vi "Main.vi"() -> ()   [LabVIEW 2021]
doc: "Use this template to build a simple state machine design pattern. Each state executes code and determines which state to transition to."
uses:
  Controls/State.ctl
  Controls/Data.ctl
  Controls/Toggle Channel.ctl
  Controls/Script Trigger Routing.ctl
  <vilib>/regexp/Match Regular Expression.xnode
  Controls/Debugging Checklist.ctl
panel:
  out "Debugging Checklist":T1
  in  "Tab Control":T2(tab)
  in  "Start Chn1 First?":bool
  in  "FGEN Resource Name":refnum<k15>
  in  "Sample Rate":dbl=20000000.0 caption="Sample Rate (Hz)" format="%#_6p"
  in  "Save Wfm List":bool
  in  "Load Wfm List":bool
  out "Waveform Preview":dbl[](graph)
  in  "Add Standard Wfm":bool
  in  "Add Custom Wfm":bool
  in  "Waveform List":i32(listbox)
  in  "Delete Selected Wfm":bool
  in  "Rename Selected Wfm":bool
  out "Total Variables":i32
  in  "Script Variable List":string[][](table) caption="Script Variable List (Editable)"
  in  "Script Trigger Routings":T3[](array[typedef])
  in  "Save Variable List":bool
  in  "Load Variable List":bool
  in  "Size to Duration":bool
  in  "Duration to Size":bool
  in  "Copy Sample Size":bool
  in  "Copy Duration":bool
  in  "Sample Size":i32
  in  "Duration (s)":dbl format="%#_6p"
  in  "Toggle Channels":T4[](array[typedef]) {"Initial State" items=["High"=101, "Low"=102]}
  in  "Start":bool
  in  "Stop":bool
  in  "Chn1 Script":string="script myScript2\n  Wait until scriptTrigger0\n  Generate Sine1kHz100us\n  Generate DcOff10us\nend script" caption="Script"
  in  "Chn0 Script":string="script myScript1\n  Generate DcOff10us\n  Generate DcOn120us marker0(tON1, tOFF1) marker1(tON2, tOFF2)\n  Generate DcOff10us\nend script" caption="Script"
  in  "Exit":bool
  # "FGEN Dual-Channel Scripts Mode Panel"
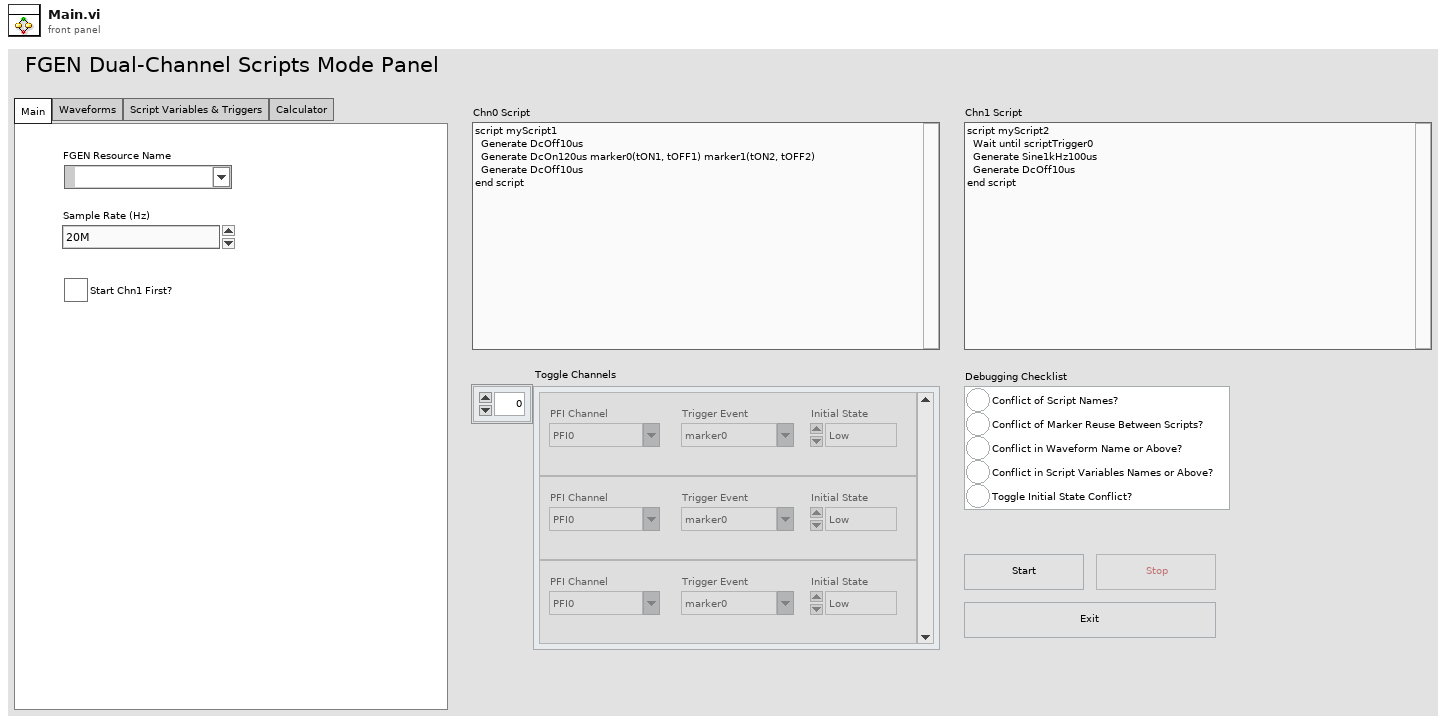
[diagram p1: front panel]
types:
  T1 = typedef "Debugging Checklist.ctl" = cluster{"Conflict of Script Names?":bool, "Conflict of Marker Reuse Between Scripts?":bool, "Conflict in Waveform Name or Above?":bool, "Conflict in Script Variables Names or Above?":bool, "Toggle Initial State Conflict?":bool}
  T2 = enum32{"Main", "Waveforms", "Script Variables & Triggers", "Calculator"}
  T3 = typedef "Script Trigger Routing.ctl" = cluster{"ID":string, "Trigger Source":string}
  T4 = typedef "Toggle Channel.ctl" = cluster{"PFI Channel":string, "Trigger Event":string, "Initial State":u16}
  T5 = typedef "Data.ctl" = cluster{"FGEN Resource Name":refnum<k15>, "Sample Rate":dbl, "Start Chn1 First?":bool, "Script Trigger Routings":T3[], "Chn0 Script":string, "Chn1 Script":string, "Toggle Channels":T4[], "Script Variable List":string[][], "Session Initialized?":bool, "Original Waveforms":waveform(dbl)[], "Chn0 Script Name":string, "Chn1 Script Name":string}
  T6 = typedef "State.ctl" = enum16{"Initialize", "Update Sample Rate", "Update Waveform List", "Update Script Variable List", "Update Scripts", "Update Toggle Channels", "Debugging Checklist", "Wait for Event", "Prepare", "Start", "Running", "Stop", "Handle Error", "Exit"}
  T7 = enum8{"Enabled", "Disabled", "Disabled and Grayed Out"}
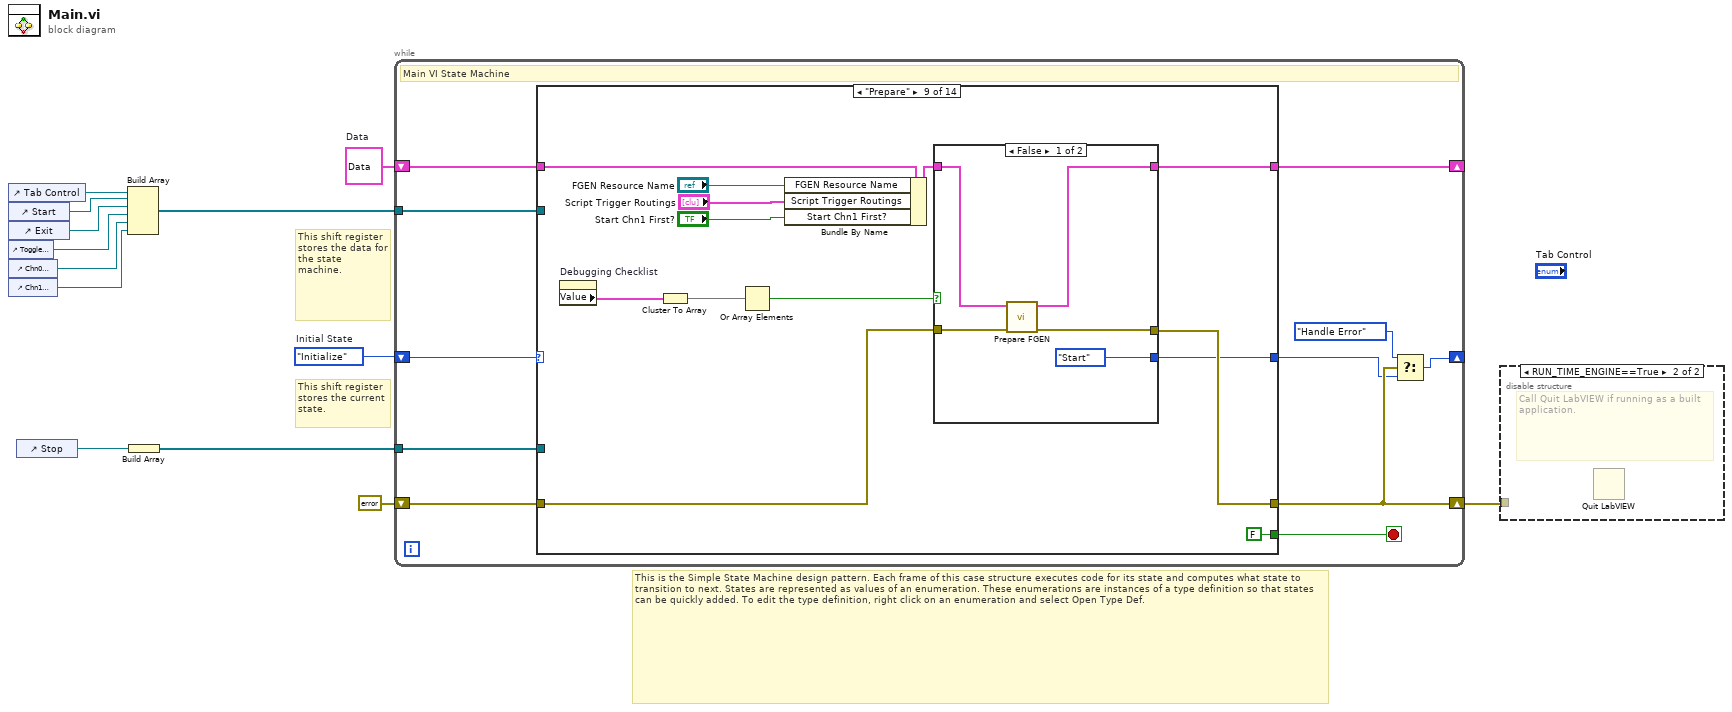
[diagram p0: block diagram]
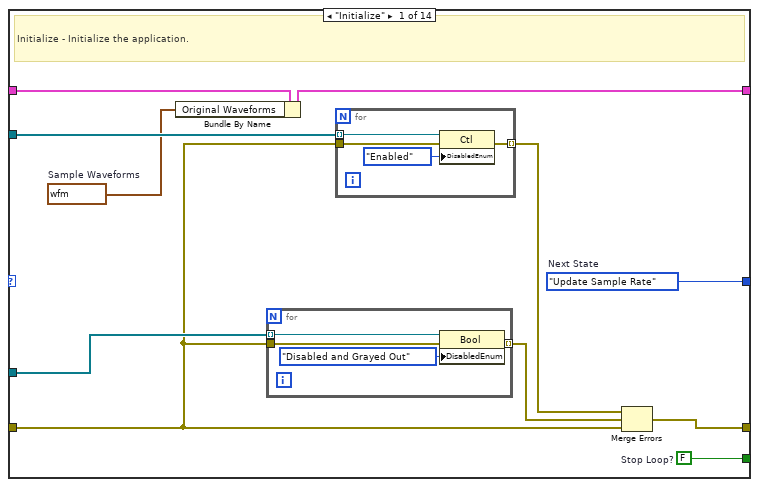
[diagram p3: hidden frame]
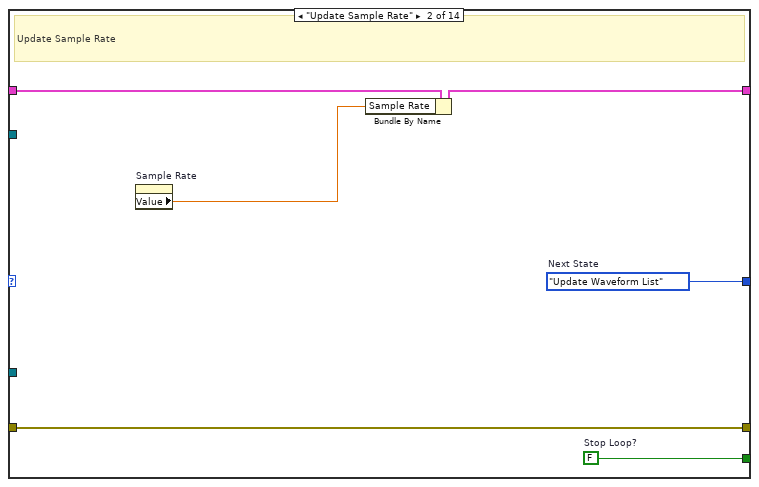
[diagram p4: hidden frame]
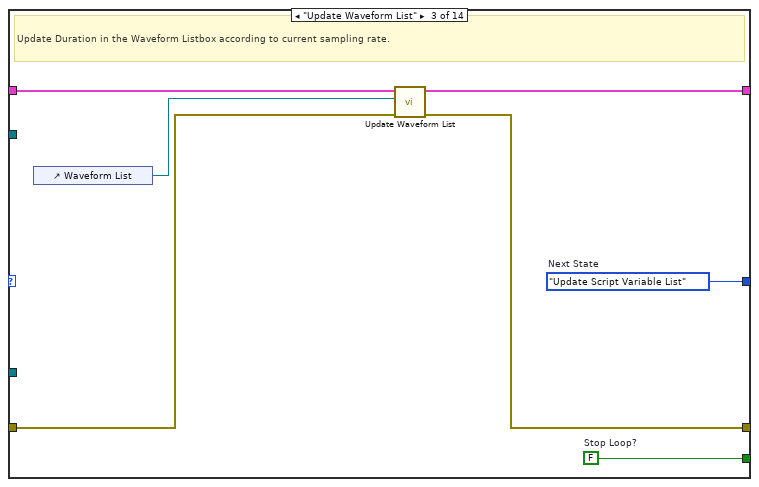
[diagram p5: hidden frame]
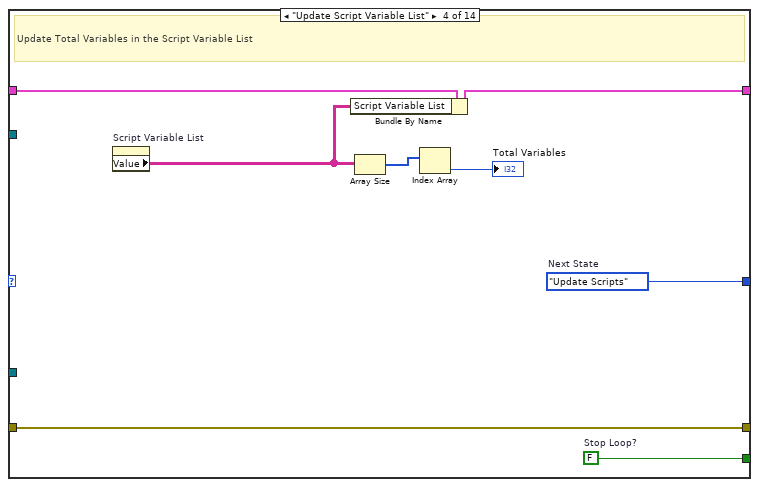
[diagram p6: hidden frame]
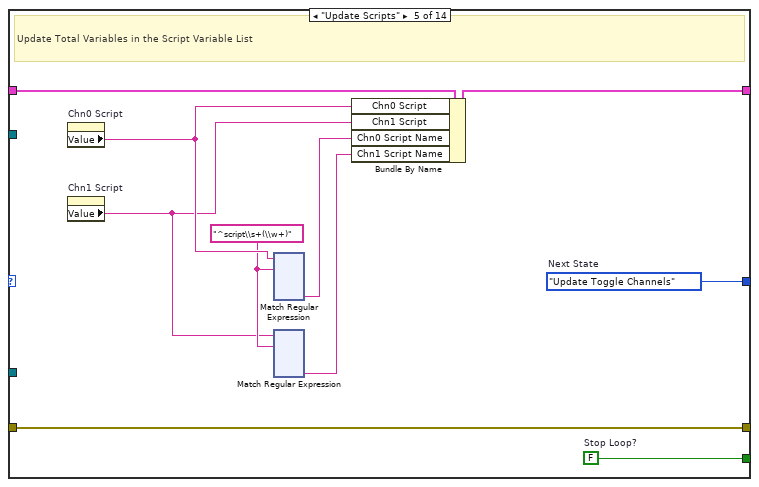
[diagram p7: hidden frame]
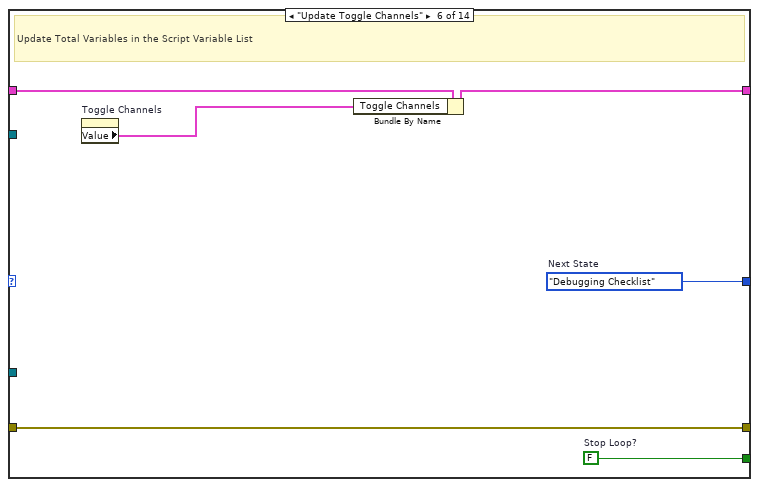
[diagram p8: hidden frame]
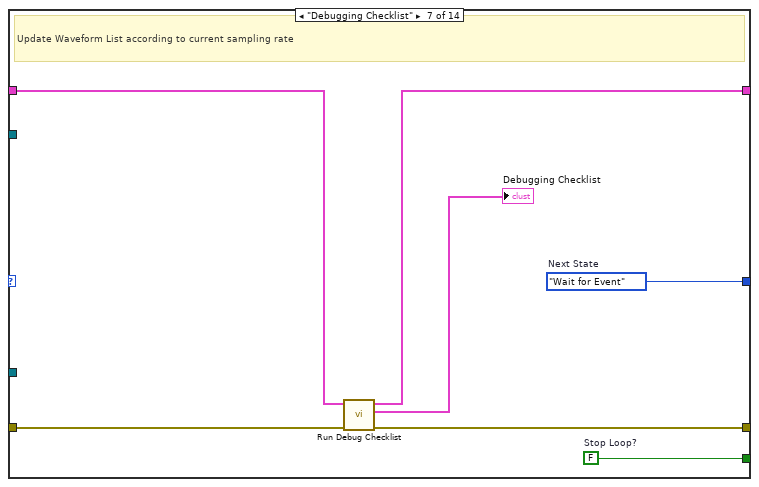
[diagram p9: hidden frame]
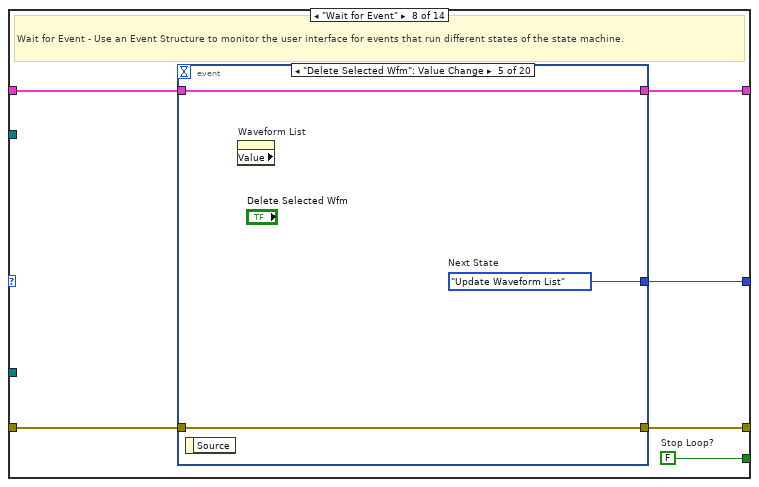
[diagram p10: hidden frame]
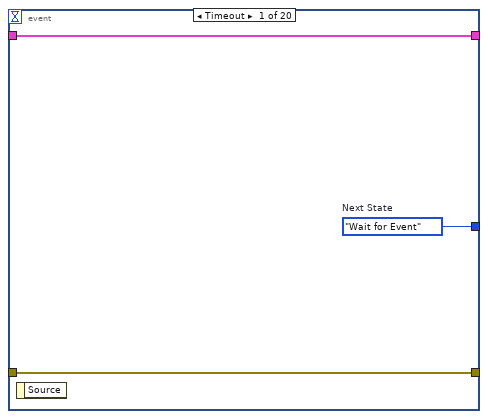
[diagram p11: hidden frame]
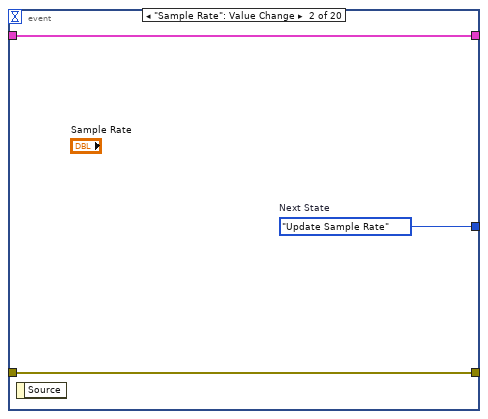
[diagram p12: hidden frame]
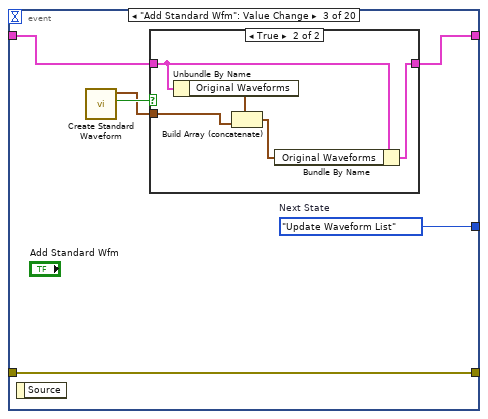
[diagram p13: hidden frame]
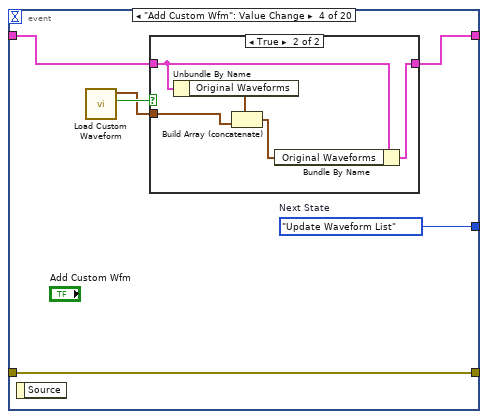
[diagram p15: hidden frame]
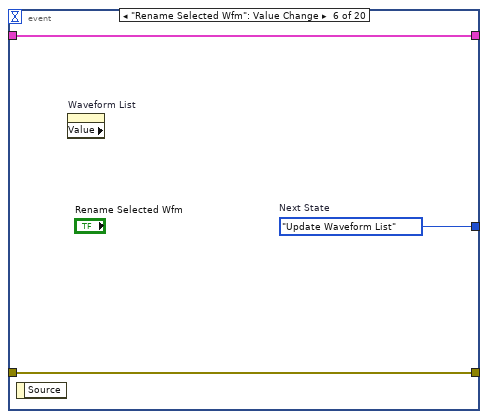
[diagram p17: hidden frame]
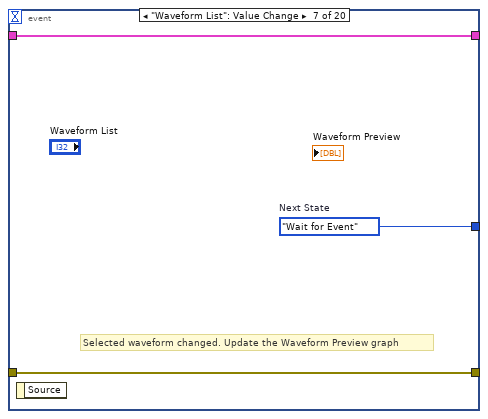
[diagram p18: hidden frame]
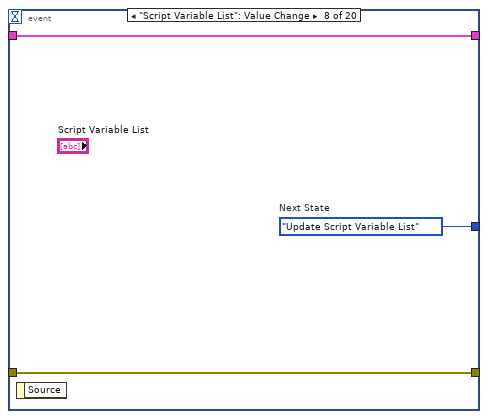
[diagram p19: hidden frame]
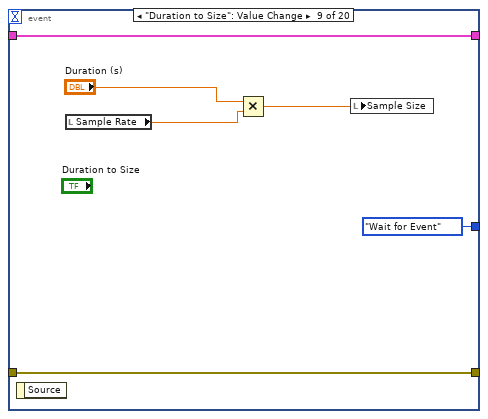
[diagram p20: hidden frame]
diagram:
  w12 = T5 {"FGEN Resource Name"="", "Sample Rate"=0.0, "Start Chn1 First?"=FALSE, "Script Trigger Routings"=[], "Chn0 Script"="", "Chn1 Script"="", "Toggle Channels"=[], "Script Variable List"=[], "Session Initialized?"=FALSE, "Original Waveforms"=[], "Chn0 Script Name"="", "Chn1 Script Name"=""}  # Data
  w13 = State."Initialize"  # Initial State
  # "This shift register stores the data for the state machine."
  # "This is the Simple State Machine design pattern. Each frame of this case structure executes code for its state and computes what state to transition to next. States are represented as values of an enumeration. These enumerations are instances of a type definition so that states can be quickly added. To edit the type definition, right click on an enumeration and select Open Type Def."
  # "This shift register stores the current state."
  n1 = control-ref of="Tab Control"() -> (w9:refnum<vi>)
  n2 = control-ref of="Start"() -> (w8:refnum<vi>)
  n3 = control-ref of="Exit"() -> (w7:refnum<vi>)
  n4 = control-ref of="Toggle Channels"() -> (w6:refnum<vi>)
  n5 = control-ref of="Chn0 Script"() -> (w5:refnum<vi>)
  n6 = control-ref of="Chn1 Script"() -> (w4:refnum<vi>)
  n7 = control-ref of="Stop"() -> (w3:refnum<vi>)
  n8 = Build Array(w9, w8, w7, w6, w5, w4) -> (w2:refnum<vi>[])
  n9 = Build Array(w3) -> (w1:refnum<vi>[])
  n10 = while {
    shift-right: [w20] -> _
    shift-left: w13 -> [w16]
    shift-right: [w23] -> _
    shift-left: w12 -> [w24]
    shift-right: [w19] -> w10
    shift-left: errorcluster {"status"=FALSE, "code"=0, "source"=""} ("error constant") -> [w22]
    tunnel: w2 -> [w14]
    tunnel: w1 -> [w15]
    stop <- w21 stop-if-true
    # "Main VI State Machine"
    n11 = case shown="\"Prepare\"" w16 {
      tunnel: [w35 w49 w56 w64 w74 w318 w325 w331 w423 State."Running" w470 State."Wait for Event" w496 w501] -> w17
      tunnel: [w34 w48 w55 w63 w73 w317 w324 w330 FALSE ("Stop Loop?") FALSE ("Stop Loop?") FALSE ("Stop Loop?") FALSE ("Stop Loop?") FALSE ("Stop Loop?") w500] -> w21
      tunnel: w24 -> [w33 w47 w52 w62 w72 w316 w320 w329 w434 w445 w465 w474 w494 w498]
      tunnel: [w26 w45 w51 w60 w70 w314 w321 w328 w432 w444 w464 w473 w494 w498] -> w23
      tunnel: w22 -> [w27 w46 w54 w61 w71 w315 w323 w327 w422 w450 w472 w479 w493 w499]
      tunnel: [w30 w46 w53 w61 w71 w315 w322 w326 w431 w449 w466 w478 w491 w499] -> w19
      tunnel: w15 -> [w31 _ _ _ _ _ _ _ _ w451 _ w480 _ _]
      tunnel: w14 -> [w32 _ _ _ _ _ _ _ _ w452 _ w481 _ _]
      frame "Initialize" {
        w25 = waveform(dbl)[] [{"t0"=timestamp(0 s since 1904-01-01), "dt"=1e-06, "Y"=[0.0, 0.0, 0.0, 0.0, 0.0, 0.0, 0.0, 0.0, 0.0, 0.0], "attributes"=variant("NI_ChannelName"=variant(string "DcOff10us"), "NI_ExpIsRelativeTime"=variant(bool TRUE), "NI_ExpStartTimeStamp"=variant(timestamp timestamp(3848638021.4949055 s since 1904-01-01)), "NI_ExpTimeStamp"=variant(timestamp timestamp(3848638021.4949055 s since 1904-01-01)), "NI_ExpXDimension"=variant(string "t"))}, {"t0"=timestamp(0 s since 1904-01-01), "dt"=1e-06, "Y"=[1.0, 1.0, 1.0, 1.0, 1.0, 1.0, 1.0, 1.0, 1.0, 1.0, 1.0, 1.0, 1.0, 1.0, 1.0, 1.0, 1.0, 1.0, 1.0, 1.0, 1.0, 1.0, 1.0, 1.0, 1.0, 1.0, 1.0, 1.0, 1.0, 1.0, 1.0, 1.0, 1.0, 1.0, 1.0, 1.0, 1.0, 1.0, 1.0, 1.0, 1.0, 1.0, 1.0, 1.0, 1.0, 1.0, 1.0, 1.0, 1.0, 1.0, 1.0, 1.0, 1.0, 1.0, 1.0, 1.0, 1.0, 1.0, 1.0, 1.0, 1.0, 1.0, 1.0, 1.0, 1.0, 1.0, 1.0, 1.0, 1.0, 1.0, 1.0, 1.0, 1.0, 1.0, 1.0, 1.0, 1.0, 1.0, 1.0, 1.0, 1.0, 1.0, 1.0, 1.0, 1.0, 1.0, 1.0, 1.0, 1.0, 1.0, 1.0, 1.0, 1.0, 1.0, 1.0, 1.0, 1.0, 1.0, 1.0, 1.0, 1.0, 1.0, 1.0, 1.0, 1.0, 1.0, 1.0, 1.0, 1.0, 1.0, 1.0, 1.0, 1.0, 1.0, 1.0, 1.0, 1.0, 1.0, 1.0, 1.0], "attributes"=variant("NI_ChannelName"=variant(string "DcOn120us"), "NI_ExpIsRelativeTime"=variant(bool TRUE), "NI_ExpStartTimeStamp"=variant(timestamp timestamp(3848638021.4959054 s since 1904-01-01)), "NI_ExpTimeStamp"=variant(timestamp timestamp(3848638021.4959054 s since 1904-01-01)), "NI_ExpXDimension"=variant(string "t"))}, {"t0"=timestamp(0 s since 1904-01-01), "dt"=5e-08, "Y"=array[2000 elements], "attributes"=variant("NI_ChannelName"=variant(string "Sine1kHz100us"), "NI_ExpIsRelativeTime"=variant(bool TRUE), "NI_ExpStartTimeStamp"=variant(timestamp timestamp(3848638021.493907 s since 1904-01-01)), "NI_ExpTimeStamp"=variant(timestamp timestamp(3848638021.493907 s since 1904-01-01)), "NI_ExpXDimension"=variant(string "t"))}]  # Sample Waveforms
        w34 = FALSE  # Stop Loop?
        w35 = State."Update Sample Rate"  # Next State
        # "Initialize - Initialize the application."
        n12 = Bundle By Name(cluster=w33, "Original Waveforms"=w25) -> (w26:T5)
        n13 = for {
          tunnel: w31 -> [w38] mode=indexing
          tunnel: [w37] -> w29 mode=indexing
          tunnel: w27 -> [w36]
          n14 = property on="Property Node" class="Bool"(reference=w38, error in=w36, "DisabledEnum"=T7."Disabled and Grayed Out" ("Disabled")) -> (error out=w37:errorcluster)  [unwired: 1 out]
        }
        n15 = for {
          tunnel: w32 -> [w42] mode=indexing
          tunnel: [w41] -> w28 mode=indexing
          tunnel: w27 -> [w40]
          n16 = property on="Property Node" class="Ctl"(reference=w42, error in=w40, "DisabledEnum"=T7."Enabled" ("Disabled")) -> (error out=w41:errorcluster)  [unwired: 1 out]
        }
        n17 = Merge Errors(w28, w29, w27) -> (w30:errorcluster)
      }
      frame "Update Sample Rate" {
        w48 = FALSE  # Stop Loop?
        w49 = State."Update Waveform List"  # Next State
        # "Update Sample Rate"
        n18 = property on="Sample Rate" class="DigNum (strict)"() -> ("Value"=w44:dbl)  [unwired: 2 in, 2 out]
        n19 = Bundle By Name(cluster=w47, "Sample Rate"=w44) -> (w45:T5)
      }
      frame "Update Waveform List" {
        w55 = FALSE  # Stop Loop?
        w56 = State."Update Script Variable List"  # Next State
        # "Update Duration in the Waveform Listbox according to current sampling rate."
        n20 = control-ref of="Waveform List"() -> (w50:refnum<vi>)
        n21 = call "Update Waveform List.vi"("error in (no error)"=w54, "Waveform Listbox Ref"=w50, "Data In"=w52) -> ("error out"=w53:errorcluster, "Data Out"=w51:T5)  [unwired: 7 in]
      }
      frame "Update Script Variable List" {
        w63 = FALSE  # Stop Loop?
        w64 = State."Update Scripts"  # Next State
        # "Update Total Variables in the Script Variable List"
        n22 = property on="Script Variable List" class="Tbl (strict)"() -> ("Value"=w59:string[][])  [unwired: 2 in, 2 out]
        n23 = Bundle By Name(cluster=w62, "Script Variable List"=w59) -> (w60:T5)
        n24 = Array Size(array=w59) -> (size(s)=w58:i32[])
        n25 = Index Array(array=w58) -> (element=→"Total Variables":i32)  [unwired: 1 in]
      }
      frame "Update Scripts" {
        w67 = "^script\\s+(\\w+)" ("regular expression")
        w73 = FALSE  # Stop Loop?
        w74 = State."Update Toggle Channels"  # Next State
        # "Update Total Variables in the Script Variable List"
        n26 = property on="Chn0 Script" class="Str"() -> ("Value"=w69:string)  [unwired: 2 in, 2 out]
        n27 = property on="Chn1 Script" class="Str"() -> ("Value"=w66:string)  [unwired: 2 in, 2 out]
        n28 = xnode "Match Regular Expression"("input string"=w69, "regular expression"=w67) -> ("submatch 1"=w68:string)  [unwired: 4 in, 5 out]
        n29 = xnode "Match Regular Expression"("input string"=w66, "regular expression"=w67) -> ("submatch 1"=w65:string)  [unwired: 4 in, 5 out]
        n30 = Bundle By Name(cluster=w72, "Chn0 Script"=w69, "Chn1 Script"=w66, "Chn0 Script Name"=w68, "Chn1 Script Name"=w65) -> (w70:T5)
      }
      frame "Update Toggle Channels" {
        w317 = FALSE  # Stop Loop?
        w318 = State."Debugging Checklist"  # Next State
        # "Update Total Variables in the Script Variable List"
        n31 = property on="Toggle Channels" class="Arr (strict)"() -> ("Value"=w313:T4[])  [unwired: 2 in, 2 out]
        n32 = Bundle By Name(cluster=w316, "Toggle Channels"=w313) -> (w314:T5)
      }
      frame "Debugging Checklist" {
        w324 = FALSE  # Stop Loop?
        w325 = State."Wait for Event"  # Next State
        # "Update Waveform List according to current sampling rate"
        n33 = call "Run Debug Checklist.vi"("error in (no error)"=w323, "Data In"=w320) -> ("error out"=w322:errorcluster, "Debugging Checklist"=→"Debugging Checklist":T1, "Data Out"=w321:T5)  [unwired: 7 in]
      }
      frame "Wait for Event" {
        w330 = FALSE  # Stop Loop?
        # "Wait for Event - Use an Event Structure to monitor the user interface for events that run different states of the state machine."
        n34 = event shown="[4] \"Delete Selected Wfm\": Value Change" {
          selector: _ -> [_ _ _ _ _ _ _ _ _ _ _ _ _ _ _ _ _ _ _ _]
          dyn-events: _ -> [_ _ _ _ _ _ _ _ _ _ _ _ _ _ _ _ _ _ _ _]
          timeout: _ -> [_ _ _ _ _ _ _ _ _ _ _ _ _ _ _ _ _ _ _ _]
          tunnel: [w332 w335 w342 w354 w362 w365 w368 w371 State."Wait for Event" ("Next State") State."Wait for Event" ("Next State") State."Wait for Event" ("Next State") State."Wait for Event" ("Next State") State."Debugging Checklist" ("Next State") State."Debugging Checklist" ("Next State") State."Update Waveform List" ("Next State") State."Wait for Event" ("Next State") State."Update Script Variable List" ("Next State") State."Wait for Event" ("Next State") State."Prepare" ("Next State") w421] -> w331
          tunnel: w329 -> [w334 w337 w341 w353 w364 w367 w370 w373 w379 w385 w391 w397 w400 w403 w406 w409 w412 w415 w418 w420]
          tunnel: [w334 w337 w340 w352 w364 w367 w370 w373 w379 w385 w391 w397 w400 w403 w406 w409 w412 w415 w418 w420] -> w328
          tunnel: w327 -> [w333 w336 w343 w355 w363 w366 w369 w372 w378 w384 w390 w396 w399 w402 w405 w408 w411 w414 w417 w419]
          tunnel: [w333 w336 w343 w355 w363 w366 w369 w372 w378 w384 w390 w396 w399 w402 w405 w408 w411 w414 w417 w419] -> w326
          event Timeout {
            w332 = State."Wait for Event"  # Next State
            n35 = event-data() -> ()  [unwired: 1 in, 1 out]
          }
          event "Sample Rate": Value Change {
            w335 = State."Update Sample Rate"  # Next State
            n36 = event-data() -> ()  [unwired: 1 in, 1 out]
          }
          event "Add Standard Wfm": Value Change {
            w342 = State."Update Waveform List"  # Next State
            n37 = event-data() -> ()  [unwired: 1 in, 1 out]
            n38 = call "Create Standard Waveform.vi"() -> ("Waveform Created?"=w339:bool, "Output Waveform"=w338:waveform(dbl))  [unwired: 10 in]
            n39 = case shown="True" w339 {
              tunnel: w341 -> [w344 w349]
              tunnel: [w344 w345] -> w340
              tunnel: w338 -> [_ w347]
              frame False {
              }
              frame True {
                n40 = Unbundle By Name(w349) -> ("Original Waveforms"=w348:waveform(dbl)[])
                n41 = Build Array (concatenate)(w348, w347) -> (w346:waveform(dbl)[])
                n42 = Bundle By Name(cluster=w349, "Original Waveforms"=w346) -> (w345:T5)
              }
            }
          }
          event "Add Custom Wfm": Value Change {
            w354 = State."Update Waveform List"  # Next State
            n43 = event-data() -> ()  [unwired: 1 in, 1 out]
            n44 = call "Load Custom Waveform.vi"() -> ("Waveform Created?"=w351:bool, "Output Waveform"=w350:waveform(dbl))  [unwired: 10 in]
            n45 = case shown="True" w351 {
              tunnel: w353 -> [w356 w361]
              tunnel: [w356 w357] -> w352
              tunnel: w350 -> [_ w359]
              frame False {
              }
              frame True {
                n46 = Unbundle By Name(w361) -> ("Original Waveforms"=w360:waveform(dbl)[])
                n47 = Build Array (concatenate)(w360, w359) -> (w358:waveform(dbl)[])
                n48 = Bundle By Name(cluster=w361, "Original Waveforms"=w358) -> (w357:T5)
              }
            }
          }
          event "Delete Selected Wfm": Value Change {
            w362 = State."Update Waveform List"  # Next State
            n49 = event-data() -> ()  [unwired: 1 in, 1 out]
            n50 = property on="Waveform List" class="MCListbox (strict)" props=["Value"]() -> ()  [unwired: 2 in, 3 out]
          }
          event "Rename Selected Wfm": Value Change {
            w365 = State."Update Waveform List"  # Next State
            n51 = event-data() -> ()  [unwired: 1 in, 1 out]
            n52 = property on="Waveform List" class="MCListbox (strict)" props=["Value"]() -> ()  [unwired: 2 in, 3 out]
          }
          event "Waveform List": Value Change {
            w368 = State."Wait for Event"  # Next State
            # "Selected waveform changed. Update the Waveform Preview graph"
            n53 = event-data() -> ()  [unwired: 1 in, 1 out]
          }
          event "Script Variable List": Value Change {
            w371 = State."Update Script Variable List"  # Next State
            n54 = event-data() -> ()  [unwired: 1 in, 1 out]
          }
          event "Duration to Size": Value Change {
            n55 = event-data() -> ()  [unwired: 1 in, 1 out]
            n56 = local read "Sample Rate"() -> (w375:dbl)
            n57 = Multiply(x="Duration (s)", y=w375) -> (x*y=w374:dbl)
            n58 = local write "Sample Size"(w374) -> ()
          }
          event "Size to Duration": Value Change {
            n59 = event-data() -> ()  [unwired: 1 in, 1 out]
            n60 = local read "Sample Rate"() -> (w382:dbl)
            n61 = Divide(x="Sample Size", y=w382) -> (x/y=w381:dbl)
            n62 = local write "Duration (s)"(w381) -> ()
          }
          event "Copy Duration": Value Change {
            n63 = event-data() -> ()  [unwired: 1 in, 1 out]
            n64 = local read "Duration (s)"() -> (w389:dbl)
            n65 = Format Into String(format string="%#_6p", w389) -> (resulting string=w388:string)  [unwired: 2 in, 1 out]
            n66 = invoke class="App" method="Clipboard.Write"("Param 0"=w388) -> ()  [unwired: 3 in, 4 out]
          }
          event "Copy Sample Size": Value Change {
            n67 = event-data() -> ()  [unwired: 1 in, 1 out]
            n68 = local read "Sample Size"() -> (w395:i32)
            n69 = Format Into String(format string="%d", w395) -> (resulting string=w394:string)  [unwired: 2 in, 1 out]
            n70 = invoke class="App" method="Clipboard.Write"("Param 0"=w394) -> ()  [unwired: 3 in, 4 out]
          }
          event "Chn0 Script", "Chn1 Script": Value Change {
            n71 = event-data() -> ()  [unwired: 1 in, 1 out]
          }
          event "Toggle Channels": Value Change {
            n72 = event-data() -> ()  [unwired: 1 in, 1 out]
          }
          event "Load Wfm List": Value Change {
            n73 = event-data() -> ()  [unwired: 1 in, 1 out]
          }
          event "Save Wfm List": Value Change {
            n74 = event-data() -> ()  [unwired: 1 in, 1 out]
          }
          event "Load Variable List": Value Change {
            n75 = event-data() -> ()  [unwired: 1 in, 1 out]
          }
          event "Save Variable List": Value Change {
            n76 = event-data() -> ()  [unwired: 1 in, 1 out]
          }
          event "Start": Value Change {
            n77 = event-data() -> ()  [unwired: 1 in, 1 out]
          }
          event "Exit": Value Change {
            w421 = State."Exit"  # Next State
            n78 = event-data() -> ()  [unwired: 1 in, 1 out]
          }
        }
      }
      frame "Prepare" {
        n79 = property on="Debugging Checklist" class="Clust (strict)"() -> ("Value"=w426:T1)  [unwired: 2 in, 2 out]
        n80 = Cluster To Array(cluster=w426) -> (array=w425:bool[])
        n81 = Or Array Elements(Boolean array=w425) -> (logical OR=w424:bool)
        n82 = Bundle By Name(cluster=w434, "FGEN Resource Name"="FGEN Resource Name", "Script Trigger Routings"="Script Trigger Routings", "Start Chn1 First?"="Start Chn1 First?") -> (w430:T5)
        n83 = case shown="False" w424 {
          tunnel: [w439 w440] -> w432
          tunnel: w422 -> [w438 w441]
          tunnel: [w437 w441] -> w431
          tunnel: w430 -> [w436 w440]
          tunnel: [State."Start" State."Wait for Event"] -> w423
          frame False {
            n84 = call "Prepare FGEN.vi"("error in (no error)"=w438, "Data In"=w436) -> ("error out"=w437:errorcluster, "Data Out"=w439:T5)  [unwired: 8 in]
          }
          frame True {
            n85 = One Button Dialog(message="Please check the Debug Checklist and fix the issue.") -> ()  [unwired: 1 in, 1 out]
          }
        }
      }
      frame "Start" {
        n86 = call "Start FGEN.vi"("error in (no error)"=w450, "Data In"=w445) -> ("error out"=w446:errorcluster, "Data Out"=w444:T5)  [unwired: 8 in]
        n87 = for {
          tunnel: w452 -> [w457] mode=indexing
          tunnel: w446 -> [w456]
          tunnel: [w455] -> w447 mode=indexing
          n88 = property on="Property Node" class="Ctl"(reference=w457, error in=w456, "DisabledEnum"=T7."Disabled and Grayed Out" ("Disabled")) -> (error out=w455:errorcluster)  [unwired: 1 out]
        }
        n89 = for {
          tunnel: w451 -> [w460] mode=indexing
          tunnel: [w459] -> w448 mode=indexing
          n90 = property on="Property Node" class="Bool"(reference=w460, "DisabledEnum"=T7."Enabled" ("Disabled")) -> (error out=w459:errorcluster)  [unwired: 1 in, 1 out]
        }
        n91 = Merge Errors(w447, w448, w446) -> (w449:errorcluster)
      }
      frame "Running" {
        # "Running until generation finish or user press Stop."
        n92 = call "Check Running FGEN.vi"("error in (no error)"=w472, "Data In"=w465) -> ("error out"=w466:errorcluster, "Done Generation"=w462:bool, "Data Out"=w464:T5)  [unwired: 7 in]
        n93 = Or(x=w462, y="Stop") -> (x .or. y?=w463:bool)
        n94 = Select(t=State."Stop", s=w463, f=State."Running") -> (s? t:f=w470:T6)
      }
      frame "Stop" {
        # "Stop FGEN if session is initialized"
        n95 = call "Stop FGEN.vi"("error in (no error)"=w479, "Data In"=w474) -> ("error out"=w475:errorcluster, "Data Out"=w473:T5)  [unwired: 8 in]
        n96 = for {
          tunnel: w481 -> [w486] mode=indexing
          tunnel: w475 -> [w485]
          tunnel: [w484] -> w476 mode=indexing
          n97 = property on="Property Node" class="Ctl"(reference=w486, error in=w485, "DisabledEnum"=T7."Enabled" ("Disabled")) -> (error out=w484:errorcluster)  [unwired: 1 out]
        }
        n98 = for {
          tunnel: w480 -> [w489] mode=indexing
          tunnel: [w488] -> w477 mode=indexing
          n99 = property on="Property Node" class="Bool"(reference=w489, "DisabledEnum"=T7."Disabled and Grayed Out" ("Disabled")) -> (error out=w488:errorcluster)  [unwired: 1 in, 1 out]
        }
        n100 = Merge Errors(w476, w477, w475) -> (w478:errorcluster)
      }
      frame "Handle Error" {
        w496 = State."Stop"  # Next State
        # "Display error message and clear it. Stop and close FGEN if needed."
        n101 = call <vilib>:"Simple Error Handler.vi"("error in (no error)"=w493) -> ("error out"=w492:errorcluster)  [unwired: 4 in, 4 out]
        n102 = call <vilib>:"Clear Errors.vi"("error in (no error)"=w492) -> ("error out"=w491:errorcluster)  [unwired: 5 in, 1 out]
      }
      frame "Exit", Default {
        w500 = TRUE  # Stop Loop?
        # "Exit - Exit the application."
        n103 = Unbundle By Name(w498) -> ("Session Initialized?"=w497:bool)
        n104 = case shown="True" w497 {
          tunnel: [State."Stop" State."Exit"] -> w501
          frame True {
            n105 = One Button Dialog(message="Session is not closed. Attempting closing. Please try again to exit.") -> ()  [unwired: 1 in, 1 out]
          }
          frame False {
          }
        }
      }
    }
    n106 = Select(t=State."Handle Error", s=w19, f=w17) -> (s? t:f=w20:T6)
  }
  n107 = disable-structure shown="RUN_TIME_ENGINE==True" {
    disable-tunnel: w10 -> [_ _]
    frame condition #0 (active) {
    }
    frame condition #1 {
      # "Call Quit LabVIEW if running as a built application."
      n108 = Quit LabVIEW() -> ()  [unwired: 1 in]
    }
  }
